vi "测试2.vi"() -> ()   [LabVIEW 2014]
panel:
  in  "主摄像头":refnum<k7>(container)
  in  "焦距缩进":bool
  in  "AXCont引用句柄":refnum<vi>
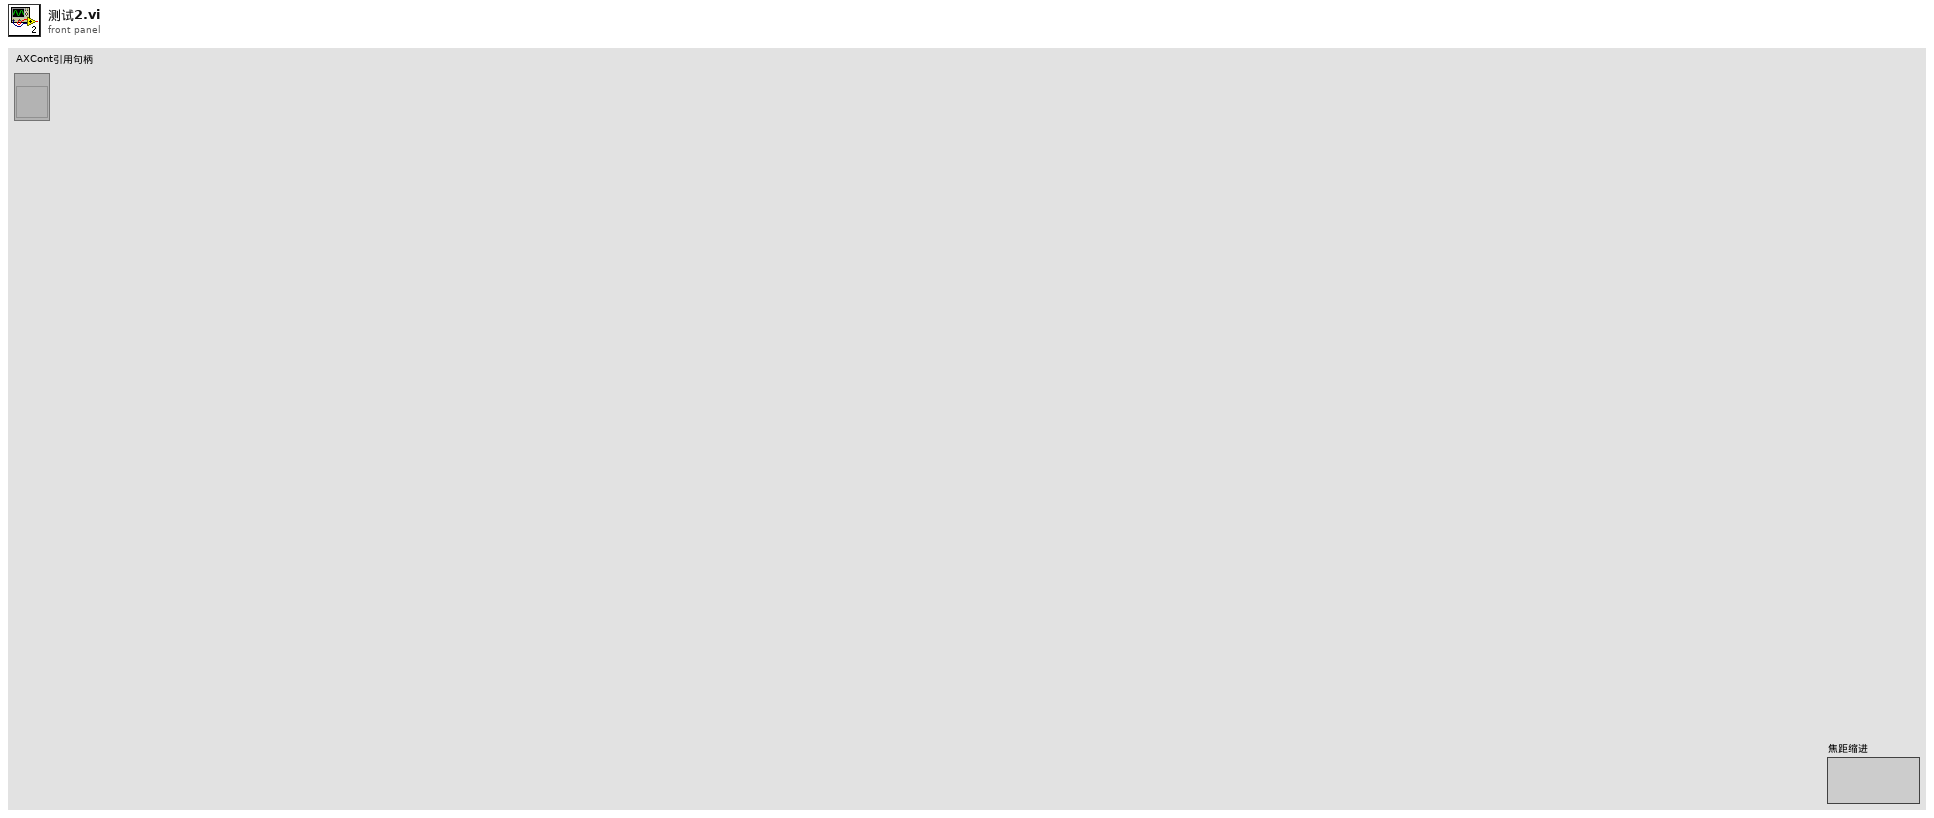
[diagram p1: front panel]
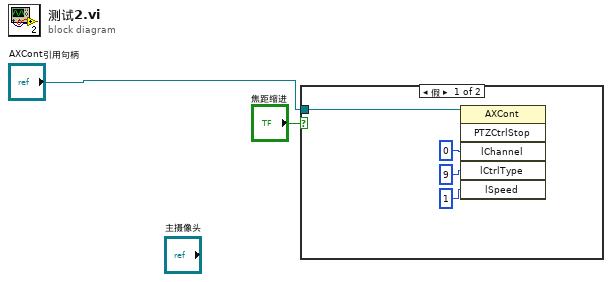
[diagram p0: block diagram]
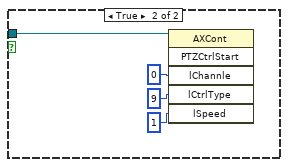
[diagram p2: hidden frame]
diagram:
  n1 = case shown="假" "焦距缩进" {
    tunnel: "AXCont引用句柄" -> [w3 w7]
    frame False {
      n2 = invoke class="AXCont" method="PTZCtrlStop"(reference=w3, "lChannel"=0, "lCtrlType"=9, "lSpeed"=1) -> ()  [unwired: 2 in, 6 out]
    }
    frame True {
      n3 = invoke class="AXCont" method="PTZCtrlStart"(reference=w7, "lChannle"=0, "lCtrlType"=9, "lSpeed"=1) -> ()  [unwired: 2 in, 6 out]
    }
  }
